vi "Configure 3 mA Chan.vi"(8 "error In":errorcluster, 10 "Output Level (1.0 mA)":dbl, 11 "VISA resource name in":refnum<visa-resource-name>) -> (0 "error out":errorcluster, 1 "Voltage":dbl format="%0.2f", 2 "Actual mA Out":dbl format="%.5f", 3 "VISA resource name out":refnum<visa-resource-name>)   [LabVIEW 2018, in "Agilent U2722.lvlib"]
uses:
  U2722 LabVIEW Instr Driver and Examples/Agilent U2722.lvlib
  <vilib>/Analysis/baseanly.llb/Mean (DBL).vi
  <vilib>/Analysis/NI_AALBase.lvlib
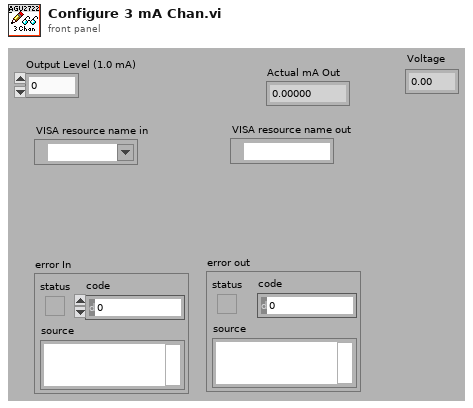
[diagram p1: front panel]
types:
  T1 = cluster{"mA Level":dbl, "Enabled?":bool, "Current Range (0: 1 uA)":u16, "Channel (1: Channel 1)":u16}[]
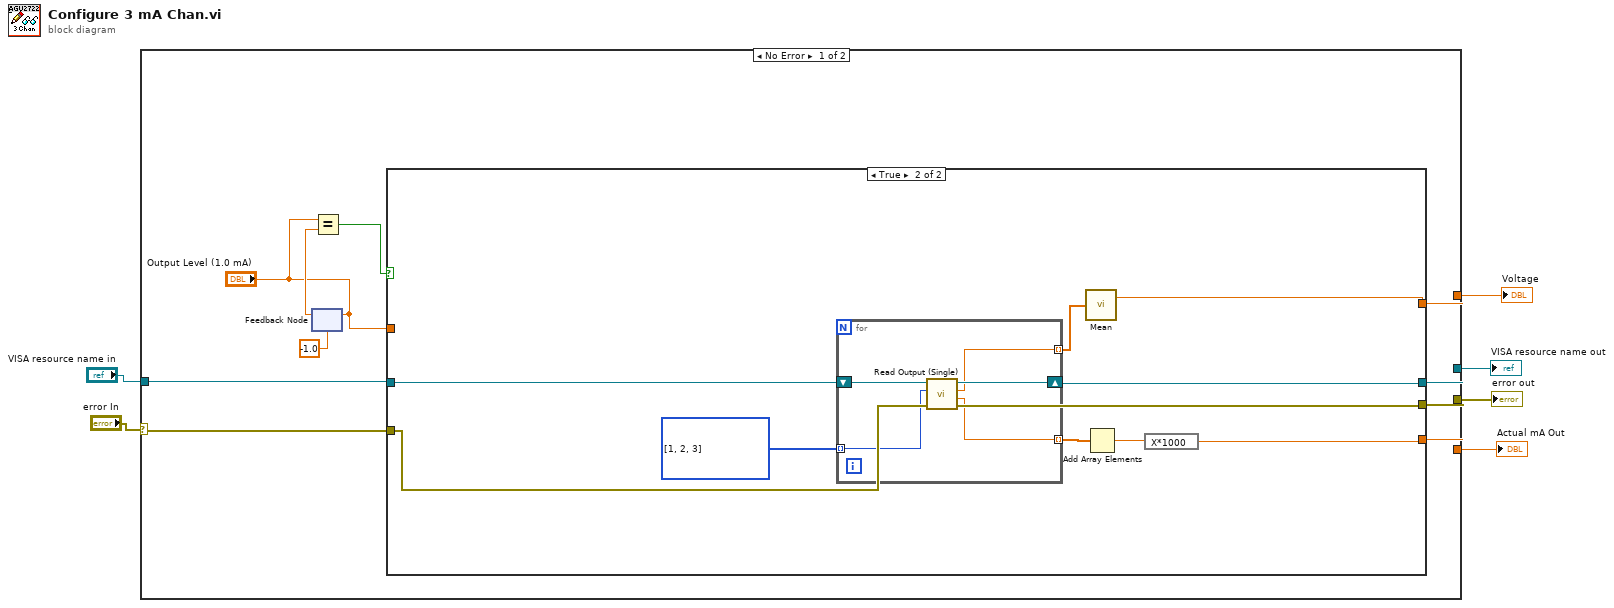
[diagram p0: block diagram]
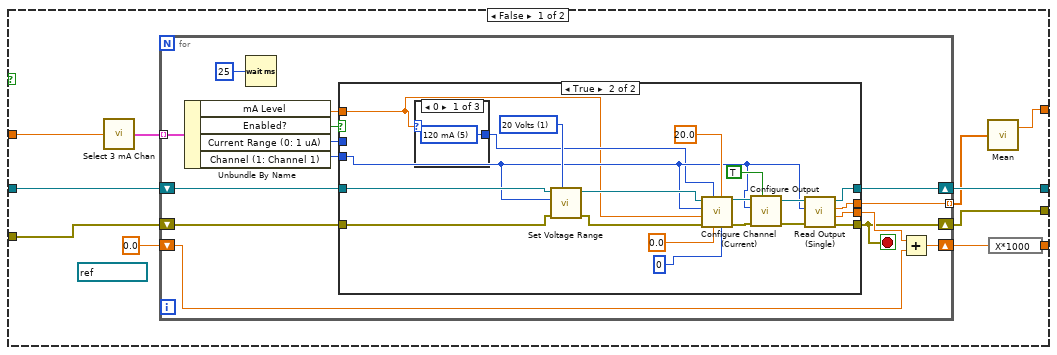
[diagram p2: hidden frame]
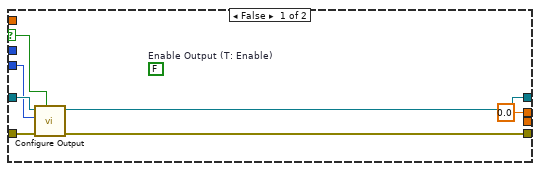
[diagram p3: hidden frame]
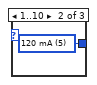
[diagram p4: hidden frame]
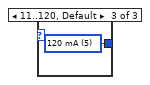
[diagram p5: hidden frame]
diagram:
  n1 = case shown="No Error" "error In" {
    selector: "error In" -> [w12 w87]
    tunnel: [w11 _] -> w5
    tunnel: [w10 _] -> w4
    tunnel: [w9 w87] -> w3
    tunnel: [w8 w86] -> w2
    tunnel: "VISA resource name in" -> [w7 w86]
    frame No Error {
      n2 = feedback #1(-1.0) -> (w15:dbl)
      n3 = feedback-in #1("Output Level (1.0 mA)") -> ()
      n4 = Equal?(x="Output Level (1.0 mA)", y=w15) -> (x = y?=w13:bool)
      n5 = case shown="True" w13 {
        tunnel: [w27 w79] -> w8
        tunnel: [w23 w73] -> w10
        tunnel: [w21 w76] -> w11
        tunnel: w7 -> [w20 w80]
        tunnel: "Output Level (1.0 mA)" -> [w19 _]
        tunnel: w12 -> [w18 w72]
        tunnel: [w17 w72] -> w9
        frame False {
          (unwired) refnum<visa-resource-name> "USB0::0x0957::0x4118::MY48130014::INSTR" ("VISA resource name in")
          n6 = call "Select 3 mA Chan.vi"("Output Level (1.0 mA)"=w19) -> ("Chan Array"=w25:T1)
          n7 = for {
            shift-right: [w30] -> w17
            shift-left: w18 -> [w40]
            shift-right: [w39] -> w27
            shift-left: w20 -> [w41]
            shift-right: [w38] -> w24
            shift-left: 0.0 -> [w37]
            tunnel: w25 -> [w36] mode=indexing
            tunnel: [w29] -> w22 mode=indexing
            stop <- w30 stop-if-true
            n8 = Unbundle By Name(w36) -> ("mA Level"=w35:dbl, "Enabled?"=w31:bool, "Current Range (0: 1 uA)"=w33:u16, "Channel (1: Channel 1)"=w34:u16)
            n9 = Wait (ms)(milliseconds to wait=u32 25) -> ()  [unwired: 1 out]
            n10 = case shown="True" w31 {
              selector: w31 -> [w44 _]
              tunnel: w41 -> [w46 w62]
              tunnel: w40 -> [w47 w60]
              tunnel: [w48 w68] -> w30
              tunnel: [w45 w67] -> w39
              tunnel: w35 -> [_ w49]
              tunnel: w34 -> [w43 w52]
              tunnel: w33 -> [_ _]
              tunnel: [_ w66] -> w32
              tunnel: [0.0 ("Actual Voltage Level (V)") w51] -> w29
              frame False {
                (unwired) FALSE  # Enable Output (T: Enable)
                n11 = call "Configure Output.vi"("Enable Output (T: Enable)"=w44, "error in (no error)"=w47, "Channel (1: Channel 1)"=w43, "VISA resource name"=w46) -> ("error out"=w48:errorcluster, "VISA resource name out"=w45:refnum<visa-resource-name>)  [unwired: 6 in]
              }
              frame True {
                w61 = u16 1 items=["2 Volts", "20 Volts"] ("Voltage Range (0: 2 Volts)")
                n12 = case shown="0" w49 {
                  tunnel: [w69 w70 w71] -> w50
                  frame 0 {
                    w69 = u16 5 items=["1 uA", "10 uA", "100 uA", "1 mA", "10 mA", "120 mA"] ("Current Range (0: 1 uA)")
                  }
                  frame 1..10 {
                    w70 = u16 5 items=["1 uA", "10 uA", "100 uA", "1 mA", "10 mA", "120 mA"] ("Current Range (0: 1 uA)")
                  }
                  frame 11..120, Default {
                    w71 = u16 5 items=["1 uA", "10 uA", "100 uA", "1 mA", "10 mA", "120 mA"] ("Current Range (0: 1 uA)")
                  }
                }
                n13 = call "Set Voltage Range.vi"("Voltage Range (0: 2 Volts)"=w61, "error in (no error)"=w60, "Channel (1: Channel 1)"=w52, "VISA resource name"=w62) -> ("error out"=w59:errorcluster, "VISA resource name out"=w58:refnum<visa-resource-name>)  [unwired: 6 in]
                n14 = call "Configure Channel (Current).vi"("Power Line Cycles (0)"=0, "Voltage Limit (2.0 V)"=20.0, "Triggered Level (1.0 mA)"=0.0, "Current Range (0: 1 uA)"=w50, "error in (no error)"=w59, "Output Level (1.0 mA)"=w49, "Channel (1: Channel 1)"=w52, "VISA resource name"=w58) -> ("error out"=w56:errorcluster, "VISA resource name out"=w57:refnum<visa-resource-name>)  [unwired: 2 in]
                n15 = call "Configure Output.vi"("Enable Output (T: Enable)"=TRUE, "error in (no error)"=w56, "Channel (1: Channel 1)"=w52, "VISA resource name"=w57) -> ("error out"=w55:errorcluster, "VISA resource name out"=w54:refnum<visa-resource-name>)  [unwired: 6 in]
                n16 = call "Read Output (Single).vi"("error in (no error)"=w55, "Channel (1: Channel 1)"=w52, "VISA resource name"=w54) -> ("error out"=w68:errorcluster, "Actual Current Level (A)"=w66:dbl, "Actual Voltage Level (V)"=w51:dbl, "VISA resource name out"=w67:refnum<visa-resource-name>)  [unwired: 5 in]
              }
            }
            n17 = Add(x=w32, y=w37) -> (x+y=w38:dbl)
          }
          n18 = call-poly <vilib>:"Mean.vi"("X"=w22) -> ("mean"=w21:dbl)  [unwired: 1 out]
          n19 = expression code="X*1000"(w24) -> (w23:dbl)
        }
        frame True {
          w78 = u16[] [1, 2, 3] items=["Channel 1"=1, "Channel 2"=2, "Channel 3"=3] ("Array")
          n20 = for {
            shift-right: [w84] -> w79
            shift-left: w80 -> [w85]
            tunnel: w78 -> [w83] mode=indexing
            tunnel: [w82] -> w77 mode=indexing
            tunnel: [w81] -> w75 mode=indexing
            n21 = call "Read Output (Single).vi"("Channel (1: Channel 1)"=w83, "VISA resource name"=w85) -> ("Actual Current Level (A)"=w81:dbl, "Actual Voltage Level (V)"=w82:dbl, "VISA resource name out"=w84:refnum<visa-resource-name>)  [unwired: 6 in, 1 out]
          }
          n22 = call-poly <vilib>:"Mean.vi"("X"=w77) -> ("mean"=w76:dbl)  [unwired: 1 out]
          n23 = Add Array Elements(numeric array=w75) -> (sum=w74:dbl)
          n24 = expression code="X*1000"(w74) -> (w73:dbl)
        }
      }
    }
    frame Error {
    }
  }
  "Voltage" <- w5
  "Actual mA Out" <- w4
  "error out" <- w3
  "VISA resource name out" <- w2
